vi "AI mnoz wartosci z przetw.vi"(8 "error in (no error)":errorcluster, 9 "A_B params in":T1, 10 "AI param aktywne in":T2[](array[typedef]) {"Numer" min=1 max=8 step=1}, 11 "Aktywne Array in":bool[](array[boolean])) -> (0 "error out":errorcluster, 1 "A_B params out":T1, 2 "AI param aktywne out":T2[](array[typedef]) {"Numer" min=1 max=8 step=1}, 3 "Aktywne Array out":bool[](array[boolean]), 4 "Mnożniki wszystkie out":dbl[](array[numeric]))   [LabVIEW 2014]
doc: "Oblicza współczynniki wielkości mierzonych\nna podstawie parametrów TransX i TransU\nprzetwornika pomiarowego"
uses:
  Kontrolki/GUI/AI_parametry.ctl
  Kontrolki/GUI/AI_typ pom.ctl
  Kontrolki/GUI/AI_wartosc.ctl
  Kontrolki/GUI/HW_A_B_params .ctl
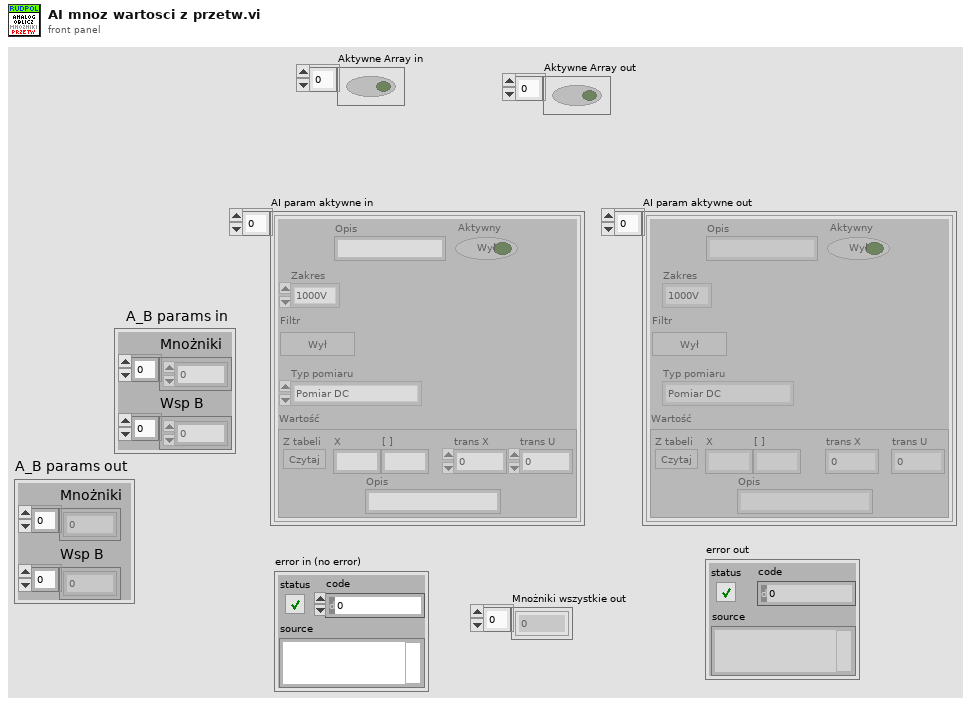
[diagram p1: front panel]
types:
  T1 = typedef "HW_A_B_params .ctl" = cluster{"Mnożniki":dbl[], "Wsp B":dbl[]}
  T2 = typedef "AI_parametry.ctl" = cluster{"Numer":u8, "Opis":string, "Zakres":enum16{"1000V", "300V", "30V", "3V", "0,3V"}, "Filtr":bool, "Typ pomiaru":T3, "Aktywny":bool, "Wartość":T4}
  T3 = typedef "AI_typ pom.ctl" = enum16{"Pomiar DC", "Pomiar AC+DC", "Pomiar AC"}
  T4 = typedef "AI_wartosc.ctl" = cluster{"X":string, "[ ]":string, "trans X":dbl, "trans U":dbl, "Z tabeli":bool, "Opis":string}
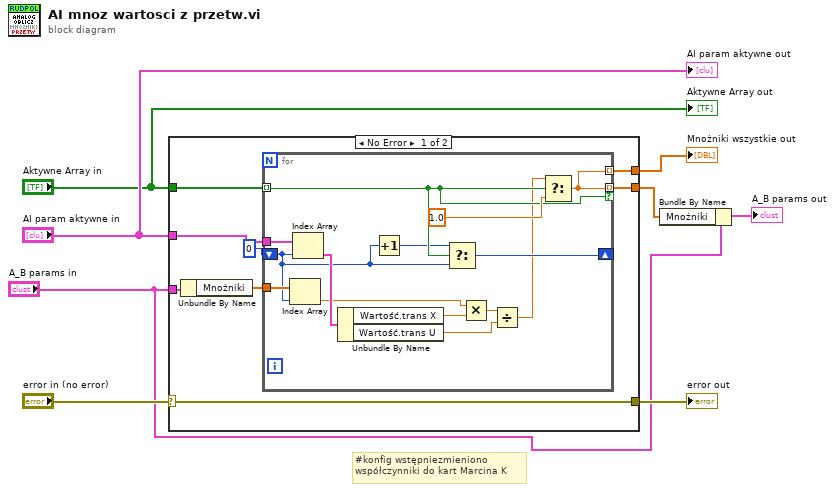
[diagram p0: block diagram]
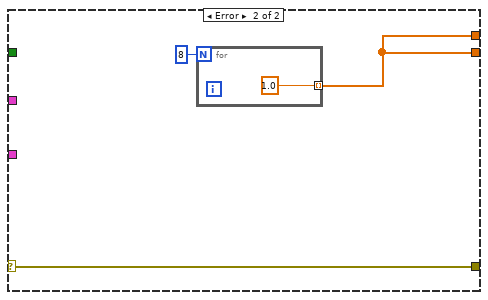
[diagram p2: hidden frame]
diagram:
  # "#konfig wstępniezmieniono\nwspółczynniki do kart Marcina K"
  n1 = case shown="No Error" "error in (no error)" {
    selector: "error in (no error)" -> [w13 w33]
    tunnel: "AI param aktywne in" -> [w15 _]
    tunnel: "Aktywne Array in" -> [w14 _]
    tunnel: [w13 w33] -> w6
    tunnel: [w12 w31] -> w1
    tunnel: [w11 w31] -> w7
    tunnel: "A_B params in" -> [w10 _]
    frame No Error {
      n2 = Unbundle By Name(w10) -> ("Mnożniki"=w9:dbl[])
      n3 = for {
        tunnel: w14 -> [w27] mode=indexing
        tunnel: w15 -> [w29]
        shift-right: [w26] -> _
        shift-left: 0 -> [w22]
        tunnel: [w24] -> w12 mode=indexing if=w27
        tunnel: [w24] -> w11 mode=indexing
        tunnel: w9 -> [w23]
        n4 = Index Array(array=w23, index=w22) -> (element=w21:dbl)
        n5 = Index Array(array=w29, index=w22) -> (element=w28:T2)
        n6 = Unbundle By Name(w28) -> ("Wartość.trans X"=w20:dbl, "Wartość.trans U"=w18:dbl)
        n7 = Increment(x=w22) -> (x+1=w25:i32)
        n8 = Select(t=w25, s=w27, f=w22) -> (s? t:f=w26:i32)
        n9 = Multiply(x=w21, y=w20) -> (x*y=w19:dbl)
        n10 = Divide(x=w19, y=w18) -> (x/y=w17:dbl)
        n11 = Select(t=w17, s=w27, f=1.0) -> (s? t:f=w24:dbl)
      }
    }
    frame Error {
      n12 = for {
        N: 8 -> [_]
        tunnel: [1.0] -> w31 mode=indexing
      }
    }
  }
  "error out" <- w6
  "Mnożniki wszystkie out" <- w7
  n13 = Bundle By Name(cluster="A_B params in", "Mnożniki"=w1) -> (→"A_B params out":T1)
  "Aktywne Array out" <- "Aktywne Array in"
  "AI param aktywne out" <- "AI param aktywne in"
